vi "Register for Process Model Notification Messages.vi"(8 "error in (no error)":errorcluster, 11 "Process Model in":refnum<class "Process Model.lvclass">) -> (0 "error out":errorcluster, 3 "Process Model out":refnum<class "Process Model.lvclass">)   [LabVIEW 2017, in "Process Model.lvlib" / "Process Model.lvclass"]
uses:
  <vilib>/gpm_packages/@cs/Car wash/Process Model/Process Model/Process Model.lvclass
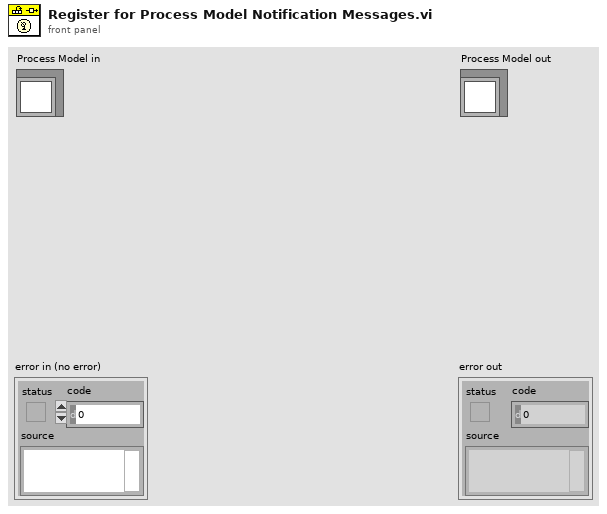
[diagram p1: front panel]
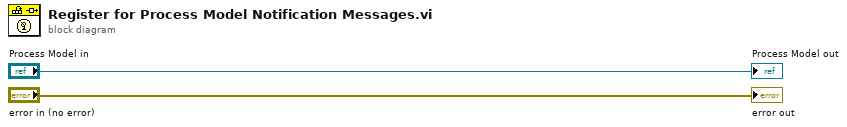
[diagram p0: block diagram]
diagram:
  "error out" <- "error in (no error)"
  "Process Model out" <- "Process Model in"
